vi "tx queue.vi"(8 "error in (no error)":errorcluster, 11 "data passing":T1) -> (0 "error out":errorcluster, 3 "data passing out":T1)   [LabVIEW 2016]
uses:
  data.ctl
  device.ctl
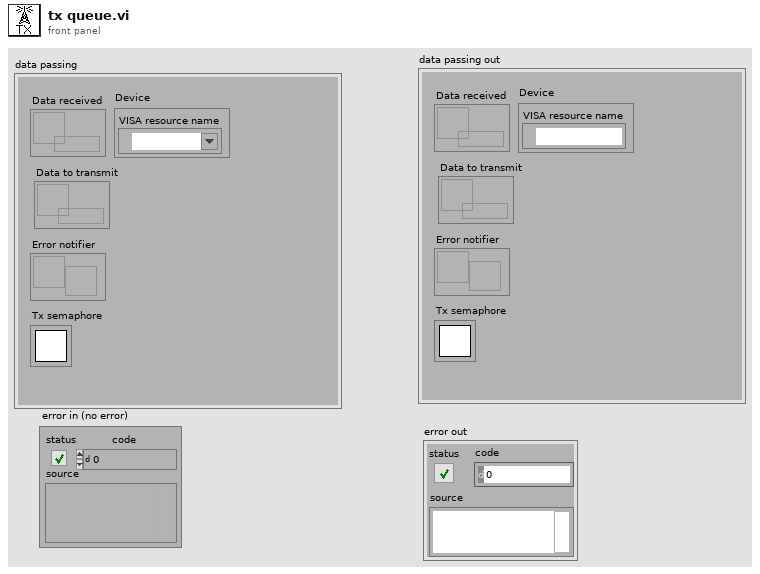
[diagram p1: front panel]
types:
  T1 = typedef "data.ctl" = cluster{"Data received":refnum<queue>, "Data to transmit":refnum<queue>, "Error notifier":refnum<notifier>, "Tx semaphore":T2, "Device":T3}
  T2 = typedef "Semaphore RefNum" = refnum<k1>
  T3 = typedef "device.ctl" = cluster{"VISA resource name":refnum<visa-resource-name>}
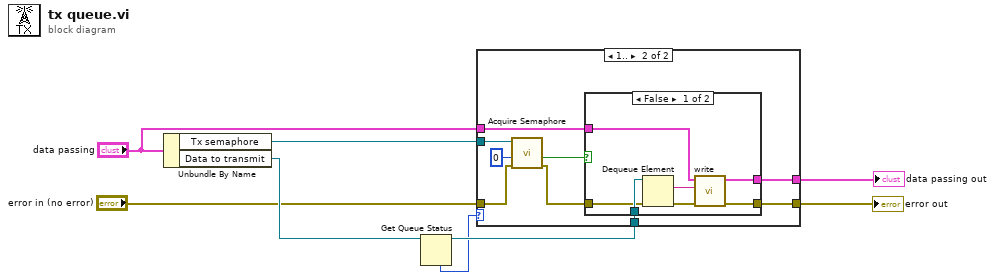
[diagram p0: block diagram]
diagram:
  n1 = Unbundle By Name("data passing") -> ("Tx semaphore"=w4:T2, "Data to transmit"=w8:refnum<queue>)
  n2 = Get Queue Status(queue=w8) -> (queue out=w6:refnum<queue>, # elements in queue=w5:i32)  [unwired: 2 in, 6 out]
  n3 = case shown="1.." w5 {
    tunnel: w6 -> [_ w19]
    tunnel: [w10 w15] -> w7
    tunnel: w4 -> [_ w14]
    tunnel: "error in (no error)" -> [w10 w13]
    tunnel: "data passing" -> [w9 w12]
    tunnel: [w9 w11] -> w1
    frame 0, Default {
    }
    frame 1.. {
      n4 = call <vilib>:"Acquire Semaphore.vi"("error in (no error)"=w13, "ms timeout (-1)"=0, "semaphore"=w14) -> ("error out"=w17:errorcluster, "timed out"=w16:bool)  [unwired: 2 in, 1 out]
      n5 = case shown="False" w16 {
        tunnel: w19 -> [w26 _]
        tunnel: w17 -> [w23 w28]
        tunnel: [w22 w28] -> w15
        tunnel: w12 -> [w21 w27]
        tunnel: [w20 w27] -> w11
        frame False {
          n6 = Dequeue Element(queue=w26, error in (no error)=w23) -> (element=w25:string, error out=w24:errorcluster)  [unwired: 1 in, 2 out]
          n7 = call "write.vi"("error in (no error)"=w24, "data"=w25, "data passing"=w21) -> ("error out"=w22:errorcluster, "data passing out"=w20:T1)  [unwired: 7 in]
        }
        frame True {
        }
      }
    }
  }
  "data passing out" <- w1
  "error out" <- w7
